vi "EMC_Contour_Move.vi"(5 "interval":dbl=0.01, 6 "points[][]":dbl[][](array[numeric]), 7 "Spline Type":i32(ring)=10682600 items=["Cubic B Spline"=10682600, "Catmull-Rom Spline"=10682601], 8 "error in (no error)":errorcluster, 9 "table":refnum<k21>, 10 "overwrite":bool, 11 "coordinate":refnum<k21>) -> (0 "error out":errorcluster)   [LabVIEW 2014]
uses:
  EMC_Typedef_Motor_Parameters.ctl
  <vilib>/Motion/PropertyNodes/nimc.createContourMoveInstance.coordinate.vi
  <vilib>/Motion/PropertyNodes/nimc.destroyInterfaceInstance.vi
  <resource>/objmgr/nimotion.rc
panel:
  in  "last update":bool
  in  "Motion Parameters":T1={"position"=1000.0, "velocity"=1000.0, "acceleration"=10000.0, "deceleration"=10000.0, "accel. jerk"=10000.0, "decel. jerk"=10000.0}
  in  "axis":refnum<k21>
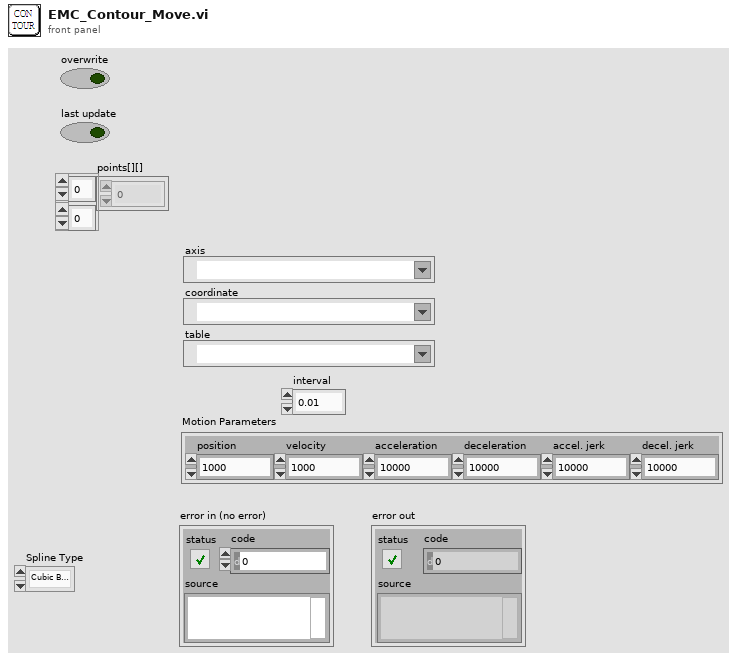
[diagram p1: front panel]
types:
  T1 = typedef "EMC_Typedef_Motor_Parameters.ctl" = cluster{"position":dbl, "velocity":dbl, "acceleration":dbl, "deceleration":dbl, "accel. jerk":dbl, "decel. jerk":dbl}
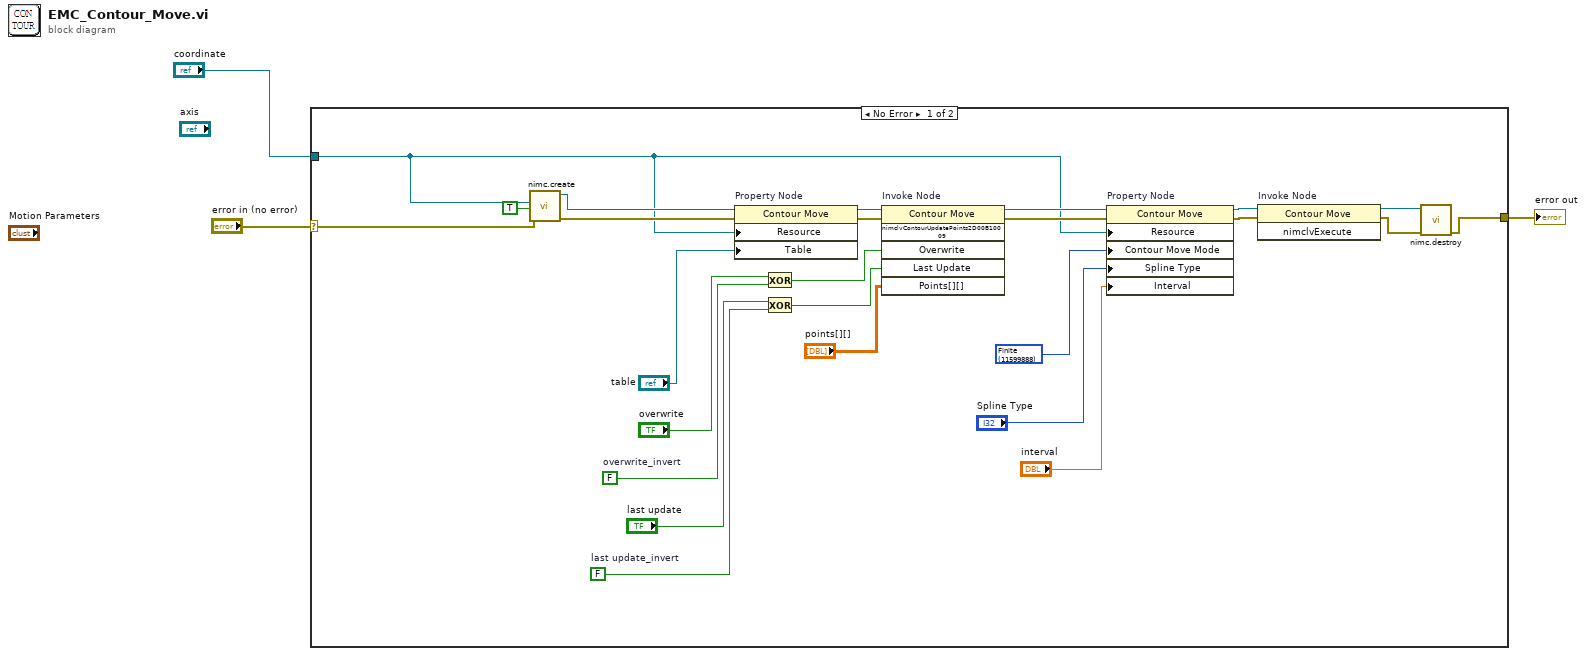
[diagram p0: block diagram]
diagram:
  n1 = case shown="No Error" "error in (no error)" {
    selector: "error in (no error)" -> [w15 w29]
    tunnel: [w6 w29] -> w2
    tunnel: "coordinate" -> [w4 _]
    frame No Error {
      w12 = 11599888 items=["Finite"=11599888, "Repetitive"=11599889, "Continuous"=11599890, "S-Curve"=11600103, "Velocity-Time"=11600111] ("contour move mode")
      w23 = FALSE  # last update_invert
      w26 = FALSE  # overwrite_invert
      n2 = call-poly <vilib>:"nimc.create.vi"("error in"=w15, "async?"=TRUE, "coordinate"=w4) -> ("error out"=w20:errorcluster, "contour"=w19:refnum<k20>)  [unwired: 6 in, 1 out]
      n3 = property on="Property Node" class="Contour Move"(reference=w19, error in=w20, "Resource"=w4, "Table"="table") -> (reference out=w18:refnum<k20>, error out=w21:errorcluster)
      n4 = Exclusive Or(1:w26, 2:"overwrite") -> (0:w27:bool)
      n5 = Exclusive Or(1:w23, 2:"last update") -> (0:w24:bool)
      n6 = invoke on="Invoke Node" class="Contour Move" method="nimclvContourUpdatePoints2D00B10009"(reference=w18, error in=w21, "Overwrite"=w27, "Last Update"=w24, "Points[][]"="points[][]") -> (reference out=w9:refnum<k20>, error out=w10:errorcluster)  [unwired: 1 in, 4 out]
      n7 = property on="Property Node" class="Contour Move"(reference=w9, error in=w10, "Resource"=w4, "Contour Move Mode"=w12, "Spline Type"="Spline Type", "Interval"="interval") -> (reference out=w13:refnum<k20>, error out=w14:errorcluster)
      n8 = invoke on="Invoke Node" class="Contour Move" method="nimclvExecute"(reference=w13, error in=w14) -> (reference out=w5:refnum<k20>, error out=w7:errorcluster)  [unwired: 1 in, 1 out]
      n9 = call-poly <vilib>:"nimc.destroy.vi"("error in"=w7, "motion handle"=w5) -> ("error out"=w6:errorcluster)  [unwired: 9 in]
    }
    frame Error {
    }
  }
  "error out" <- w2
